vi "Upload Photo.vi"(8 "Description":string="just testing", 9 "Photoset Name":string="Photobooth Testing", 10 "Image Path":string, 11 "Flickr Ref":refnum<k24>) -> (3 "Flickr Ref out":refnum<k24>)   [LabVIEW 2010]
uses:
  C:/Users/telsey/Desktop/Personal Projects/Photobooth/Flickr API/FlickrNet-3.5.0/FlickrNet.dll
  FlickrNet.dll
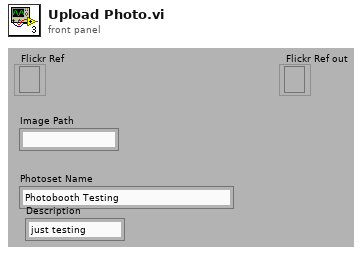
[diagram p1: front panel]
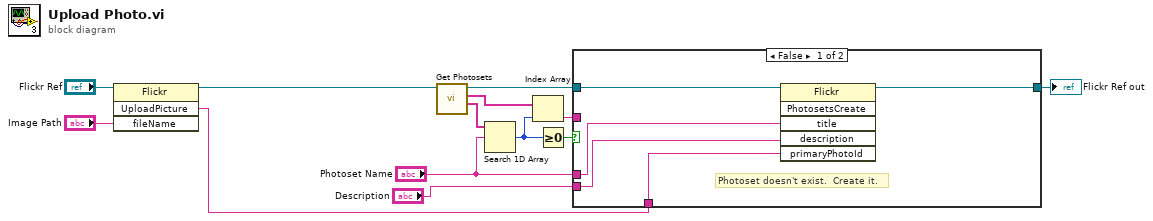
[diagram p0: block diagram]
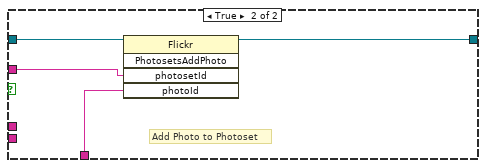
[diagram p2: hidden frame]
diagram:
  n1 = invoke class="Flickr" method="UploadPicture"(reference="Flickr Ref", "fileName"="Image Path") -> (reference out=w5:refnum<k24>, "UploadPicture"=w7:string)  [unwired: 2 in, 2 out]
  n2 = call "Get Photosets.vi"("Flickr Ref"=w5) -> ("Names"=w3:string[], "ids"=w2:string[], "Flickr Ref out"=w4:refnum<k24>)  [unwired: 8 in]
  n3 = Search 1D Array(1D array=w3, element="Photoset Name") -> (index of element=w10:i32)  [unwired: 1 in]
  n4 = Index Array(array=w2, index=w10) -> (element=w11:string)
  n5 = Greater Or Equal To 0?(x=w10) -> (x >= 0?=w9:bool)
  n6 = case shown="False" w9 {
    tunnel: w7 -> [w18 w20]
    tunnel: w4 -> [w17 w22]
    tunnel: w11 -> [_ w21]
    tunnel: [w16 w19] -> w13
    tunnel: "Photoset Name" -> [w15 _]
    tunnel: "Description" -> [w14 _]
    frame False {
      # "Photoset doesn't exist.  Create it."
      n7 = invoke class="Flickr" method="PhotosetsCreate"(reference=w17, "title"=w15, "description"=w14, "primaryPhotoId"=w18) -> (reference out=w16:refnum<k24>)  [unwired: 2 in, 5 out]
    }
    frame True {
      # "Add Photo to Photoset"
      n8 = invoke class="Flickr" method="PhotosetsAddPhoto"(reference=w22, "photosetId"=w21, "photoId"=w20) -> (reference out=w19:refnum<k24>)  [unwired: 2 in, 4 out]
    }
  }
  "Flickr Ref out" <- w13
